vi "Analysis.Build Name Lookup List, from 1D Str.vi"(11 "Unique List in":string[](array[string])) -> (3 "Lookup Out":variant)   [LabVIEW 2024]
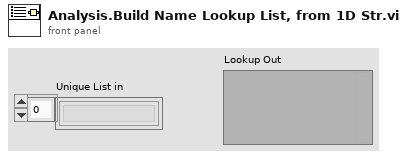
[diagram p1: front panel]
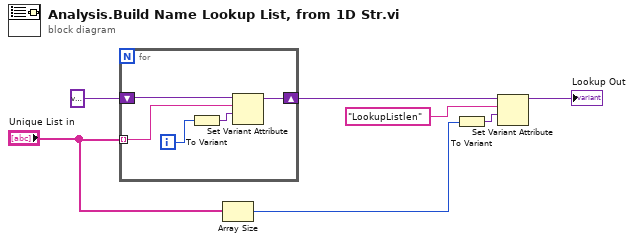
[diagram p0: block diagram]
diagram:
  n1 = for {
    tunnel: "Unique List in" -> [w11] mode=indexing
    shift-right: [w9] -> w4
    shift-left: variant -> [w12]
    i -> [w8]
    n2 = To Variant(anything=w8) -> (Variant=w10:variant)
    n3 = Set Variant Attribute(Variant=w12, name=w11, value=w10) -> (Variant out=w9:variant)  [unwired: 1 in, 2 out]
  }
  n4 = Array Size(array="Unique List in") -> (size(s)=w1:i32)
  n5 = To Variant(anything=w1) -> (Variant=w5:variant)
  n6 = Set Variant Attribute(Variant=w4, name="LookupListlen", value=w5) -> (Variant out=→"Lookup Out":variant)  [unwired: 1 in, 2 out]
